vi "Producer:Consumer_UserEvent.vi"() -> ()   [LabVIEW 2023]
panel:
  out "평가 데이터":string
  out "분석 데이터":bool
  out "측정 데이터":i32[](array[numeric])
  in  "종료":bool
  in  "평가":bool
  in  "분석":bool
  in  "측정":bool
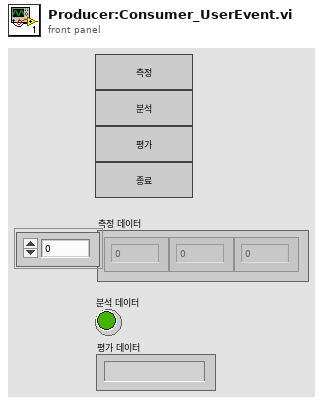
[diagram p1: front panel]
types:
  T1 = typedef "상태.ctl" = enum16{"측정", "분석", "평가", "종료"}
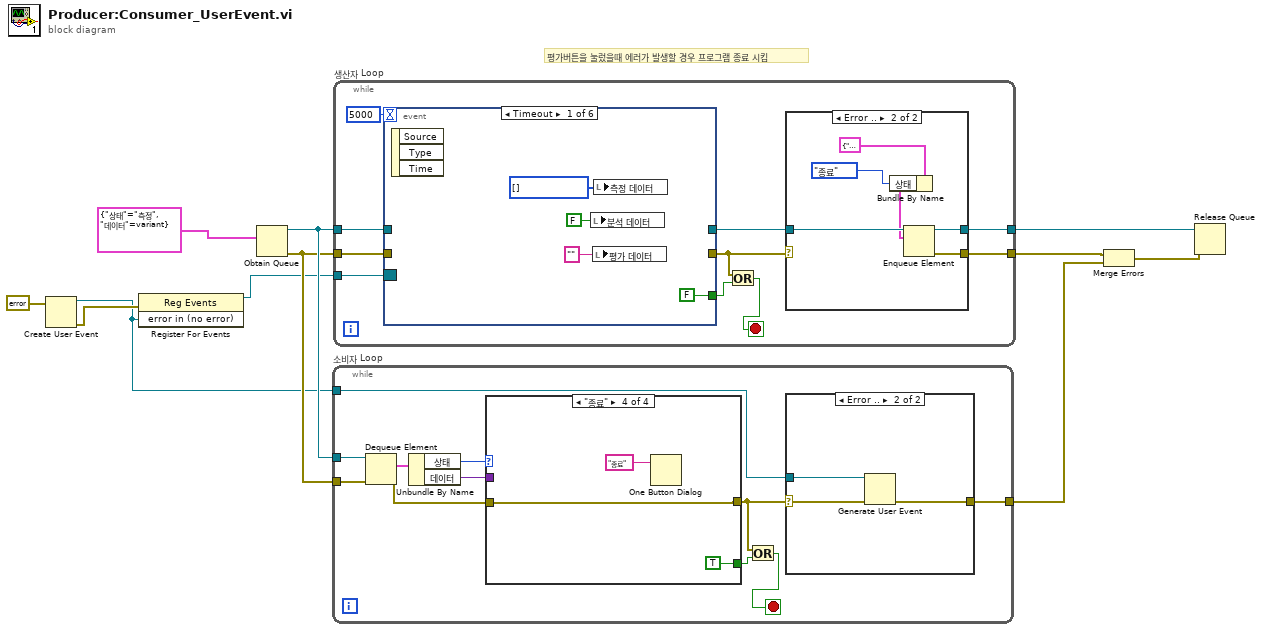
[diagram p0: block diagram]
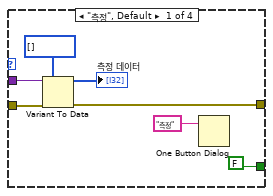
[diagram p3: hidden frame]
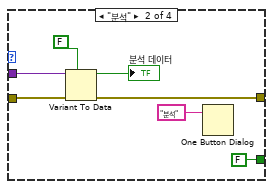
[diagram p4: hidden frame]
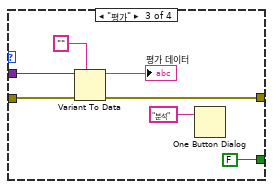
[diagram p5: hidden frame]
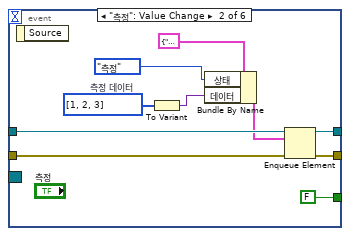
[diagram p7: hidden frame]
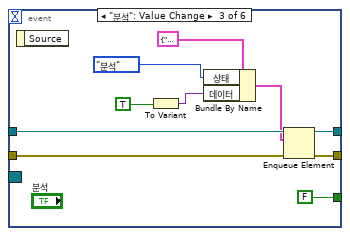
[diagram p8: hidden frame]
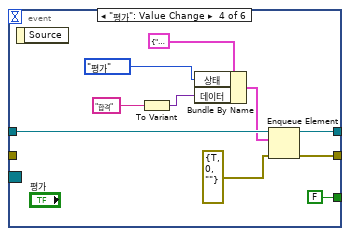
[diagram p9: hidden frame]
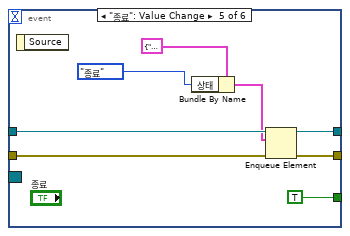
[diagram p10: hidden frame]
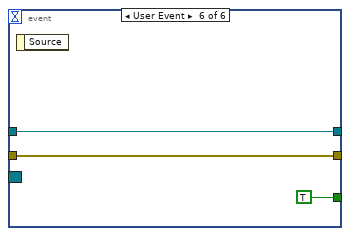
[diagram p11: hidden frame]
diagram:
  # "평가버튼을 눌렀을때 에러가 발생할 경우 프로그램 종료 시킴"
  n1 = Create User Event(user event datatype=errorcluster {"status"=FALSE, "code"=0, "source"=""} ("error in (no error)")) -> (user event=w1:refnum<user-event>, error out=w3:errorcluster)  [unwired: 1 in]
  n2 = register-events(error in=w3, w1) -> (reference out=w2:refnum<event-registration>)  [unwired: 1 in, 1 out]
  n3 = Obtain Queue(element data type=cluster{"상태":T1, "데이터":variant} {"상태"=enum."측정", "데이터"=variant}) -> (queue out=w11:refnum<queue>, error out=w10:errorcluster)  [unwired: 4 in, 1 out]
  n4 = while "소비자 Loop" {
    tunnel: w11 -> [w22]
    tunnel: w10 -> [w21]
    tunnel: [w12] -> w7
    tunnel: w1 -> [w13]
    stop <- w15 stop-if-true
    n5 = Dequeue Element(queue=w22, error in (no error)=w21) -> (element=w20:cluster{"상태":T1, "데이터":variant}, error out=w17:errorcluster)  [unwired: 1 in, 2 out]
    n6 = Unbundle By Name(w20) -> ("상태"=w19:T1, "데이터"=w18:variant)
    n7 = case shown="\"종료\"" w19 {
      tunnel: w18 -> [w33 w40 w46 _]
      tunnel: [FALSE FALSE FALSE TRUE] -> w16
      tunnel: w17 -> [w28 w35 w42 w48]
      tunnel: [w27 w34 w41 w48] -> w14
      frame "측정", Default {
        n8 = Variant To Data(error in=w28, type=i32[] [] ("측정 데이터"), Variant=w33) -> (data=→"측정 데이터":i32[], error out=w27:errorcluster)
        n9 = One Button Dialog(message="측정") -> ()  [unwired: 1 in, 1 out]
      }
      frame "분석" {
        n10 = Variant To Data(error in=w35, type=FALSE ("분석 데이터"), Variant=w40) -> (data=→"분석 데이터":bool, error out=w34:errorcluster)
        n11 = One Button Dialog(message="분석") -> ()  [unwired: 1 in, 1 out]
      }
      frame "평가" {
        n12 = Variant To Data(error in=w42, type="" ("평가 데이터"), Variant=w46) -> (data=→"평가 데이터":string, error out=w41:errorcluster)
        n13 = One Button Dialog(message="분석") -> ()  [unwired: 1 in, 1 out]
      }
      frame "종료" {
        n14 = One Button Dialog(message="종료") -> ()  [unwired: 1 in, 1 out]
      }
    }
    n15 = Or(x=w14, y=w16) -> (x .or. y?=w15:bool)
    n16 = case shown="Error .." w14 {
      selector: w14 -> [w23 w26]
      tunnel: w13 -> [_ w25]
      tunnel: [w23 w24] -> w12
      frame No Error {
      }
      frame Error {
        n17 = Generate User Event(user event=w25, event data cluster=w26) -> (error out=w24:errorcluster)  [unwired: 2 in, 1 out]
      }
    }
  }
  n18 = while "생산자 Loop" {
    tunnel: w10 -> [w60]
    tunnel: w11 -> [w59]
    tunnel: [w53] -> w6
    tunnel: [w52] -> w5
    tunnel: w2 -> [w51]
    stop <- w56 stop-if-true
    n19 = event shown="[0] Timeout" {
      selector: w51 -> [_ _ _ _ _ _]
      dyn-events: _ -> [_ _ _ _ _ _]
      timeout: 5000 -> [_ _ _ _ _ _]
      tunnel: w60 -> [_ w82 w86 _ w106 w111]
      tunnel: [_ w81 w87 w100 w105 w111] -> w55
      tunnel: w59 -> [_ w80 w89 w102 w108 w112]
      tunnel: [_ w79 w88 w101 w107 _] -> w54
      tunnel: [FALSE FALSE FALSE FALSE TRUE TRUE] -> w57
      tunnel: [_ _ _ _ _ w112] -> _
      event Timeout {
        n20 = event-data() -> ()  [unwired: 1 in, 3 out]
        n21 = local write "분석 데이터"(FALSE ("분석 데이터")) -> ()
        n22 = local write "평가 데이터"("" ("평가 데이터")) -> ()
        n23 = local write "측정 데이터"(i32[] [] ("측정 데이터")) -> ()
      }
      event "측정": Value Change {
        w75 = i32[] [1, 2, 3]  # 측정 데이터
        n24 = event-data() -> ()  [unwired: 1 in, 1 out]
        n25 = To Variant(anything=w75) -> (Variant=w76:variant)
        n26 = Bundle By Name(cluster=cluster{"상태":T1, "데이터":variant} {"상태"=enum."측정", "데이터"=variant}, "상태"=상태."측정", "데이터"=w76) -> (w74:cluster{"상태":T1, "데이터":variant})
        n27 = Enqueue Element(queue=w80, element=w74, error in (no error)=w82) -> (queue out=w79:refnum<queue>, error out=w81:errorcluster)  [unwired: 1 in, 1 out]
      }
      event "분석": Value Change {
        n28 = event-data() -> ()  [unwired: 1 in, 1 out]
        n29 = To Variant(anything=TRUE ("분석 데이터")) -> (Variant=w90:variant)
        n30 = Bundle By Name(cluster=cluster{"상태":T1, "데이터":variant} {"상태"=enum."측정", "데이터"=variant}, "상태"=상태."분석", "데이터"=w90) -> (w84:cluster{"상태":T1, "데이터":variant})
        n31 = Enqueue Element(queue=w89, element=w84, error in (no error)=w86) -> (queue out=w88:refnum<queue>, error out=w87:errorcluster)  [unwired: 1 in, 1 out]
      }
      event "평가": Value Change {
        n32 = event-data() -> ()  [unwired: 1 in, 1 out]
        n33 = To Variant(anything="합격" ("평가 데이터")) -> (Variant=w97:variant)
        n34 = Bundle By Name(cluster=cluster{"상태":T1, "데이터":variant} {"상태"=enum."측정", "데이터"=variant}, "상태"=상태."평가", "데이터"=w97) -> (w96:cluster{"상태":T1, "데이터":variant})
        n35 = Enqueue Element(queue=w102, element=w96, error in (no error)=errorcluster {"status"=TRUE, "code"=0, "source"=""}) -> (queue out=w101:refnum<queue>, error out=w100:errorcluster)  [unwired: 1 in, 1 out]
      }
      event "종료": Value Change {
        n36 = event-data() -> ()  [unwired: 1 in, 1 out]
        n37 = Bundle By Name(cluster=cluster{"상태":T1, "데이터":variant} {"상태"=enum."측정", "데이터"=variant}, "상태"=상태."종료") -> (w104:cluster{"상태":T1, "데이터":variant})
        n38 = Enqueue Element(queue=w108, element=w104, error in (no error)=w106) -> (queue out=w107:refnum<queue>, error out=w105:errorcluster)  [unwired: 1 in, 1 out]
      }
      event User Event {
        n39 = event-data() -> ()  [unwired: 1 in, 1 out]
      }
    }
    n40 = Or(x=w55, y=w57) -> (x .or. y?=w56:bool)
    n41 = case shown="Error .." w55 {
      selector: w55 -> [w61 _]
      tunnel: w54 -> [w62 w66]
      tunnel: [w62 w65] -> w53
      tunnel: [w61 w64] -> w52
      frame No Error {
      }
      frame Error {
        n42 = Bundle By Name(cluster=cluster{"상태":T1, "데이터":variant} {"상태"=enum."측정", "데이터"=variant}, "상태"=상태."종료") -> (w63:cluster{"상태":T1, "데이터":variant})
        n43 = Enqueue Element(queue=w66, element=w63) -> (queue out=w65:refnum<queue>, error out=w64:errorcluster)  [unwired: 2 in, 1 out]
      }
    }
  }
  n44 = Merge Errors(w5, w7) -> (w8:errorcluster)
  n45 = Release Queue(queue=w6, error in (no error)=w8) -> ()  [unwired: 1 in, 3 out]
